vi "StoreBinary_Local.vi"(0 "Data Array":dbl[](array[numeric]), 1 "Number of Channels":u32, 5 "Filename":string, 7 "Fname Increment":u8, 9 "Save Type":u16(ring)=1 items=["USB", "cRIO"], 11 "Bin Header":i32=2, 12 "Block Size":u32, 13 "error in (no error)":errorcluster) -> (3 "Low on Free Disk Space":bool, 4 "New Fname":string, 6 "New Save Type":u16, 8 "Current Free Space (Mb)":dbl, 10 "NewFnameCount":u8, 14 "error out":errorcluster, 15 "Counter Out":i32)   [LabVIEW 2013]
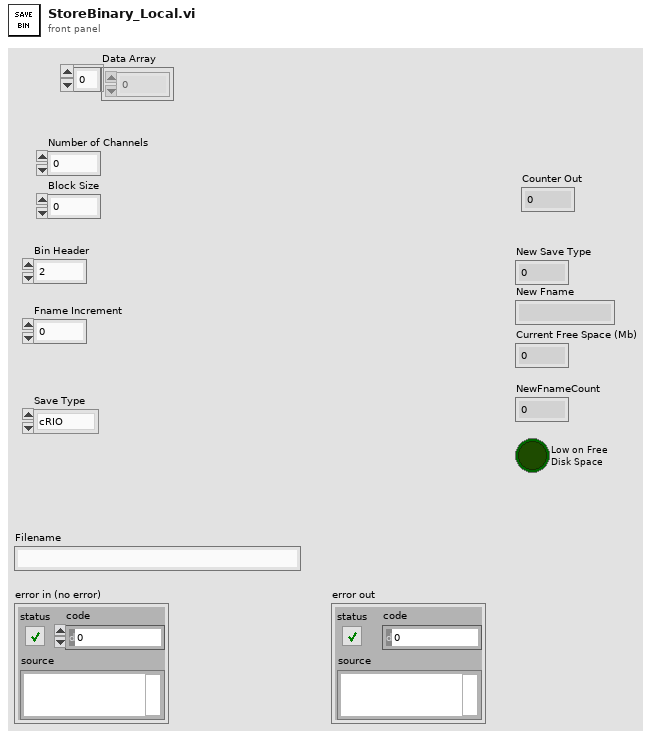
[diagram p1: front panel]
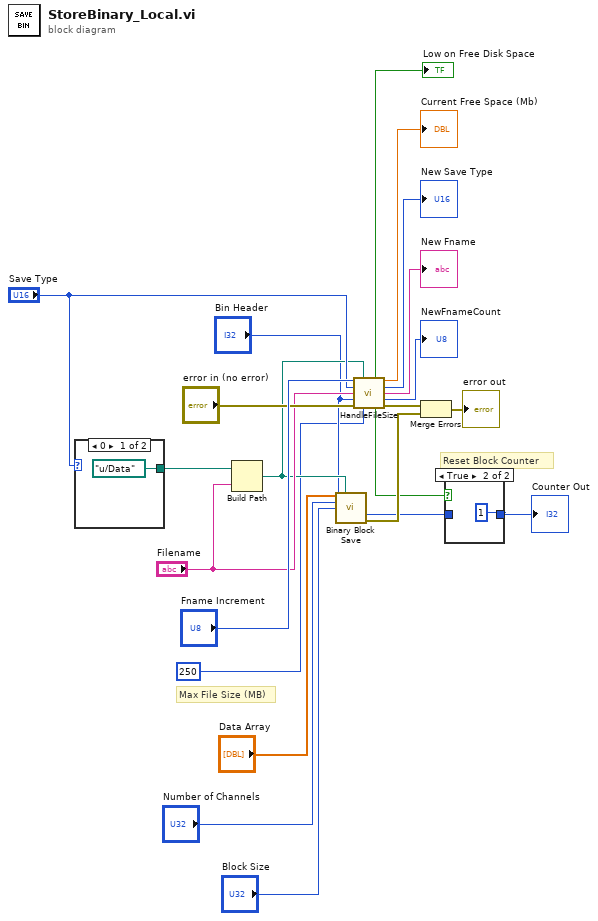
[diagram p0: block diagram]
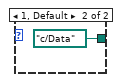
[diagram p3: hidden frame]
diagram:
  # "Max File Size (MB)"
  # "Reset Block Counter"
  n1 = case shown="0" "Save Type" {
    tunnel: [path "u:/Data" path "c:/Data"] -> w19
    frame 0 {
    }
    frame 1, Default {
    }
  }
  n2 = Build Path(base path=w19, name or relative path="Filename") -> (appended path=w10:path)
  n3 = call "Binary Block Save.vi"("Data Array"="Data Array", "file path (use dialog)"=w10, "Number of Channels"="Number of Channels", "Block Size"="Block Size", "Counter In"="Bin Header") -> ("Counter Out"=w4:i32, "error out"=w6:errorcluster)  [unwired: 9 in]
  n4 = call "HandleFileSize.vi"("FName Increment Count"="Fname Increment", "path"=w10, "Save Type"="Save Type", "Filename"="Filename", "Bin Header"="Bin Header", "error in"="error in (no error)", "Max File Size (MB)"=i64 250) -> ("Low on Free Disk Space"=→"Low on Free Disk Space":bool, "Current Free Space (Mb)"=→"Current Free Space (Mb)":dbl, "New Save Type"=→"New Save Type":u16, "New Fname"=→"New Fname":string, "NewFnameCount"=→"NewFnameCount":u8, "NewFileName Check"=w3:bool, "error out"=w7:errorcluster)  [unwired: 2 in]
  n5 = Merge Errors(w7, w6) -> (→"error out":errorcluster)
  n6 = case shown="True" w3 {
    tunnel: w4 -> [w25 _]
    tunnel: [w25 1 ("Counter Out")] -> w2
    frame False {
    }
    frame True {
    }
  }
  "Counter Out" <- w2
